vi "Read Task List.vi"(4 "Error In":errorcluster, 7 "Image Name":string) -> (0 "Error Out":errorcluster, 2 "Processes Found":i32, 3 "Processes":T1(array[cluster]))   [LabVIEW 2014, in "Managing Executables.lvlib"]
uses:
  Managing Executables.lvlib
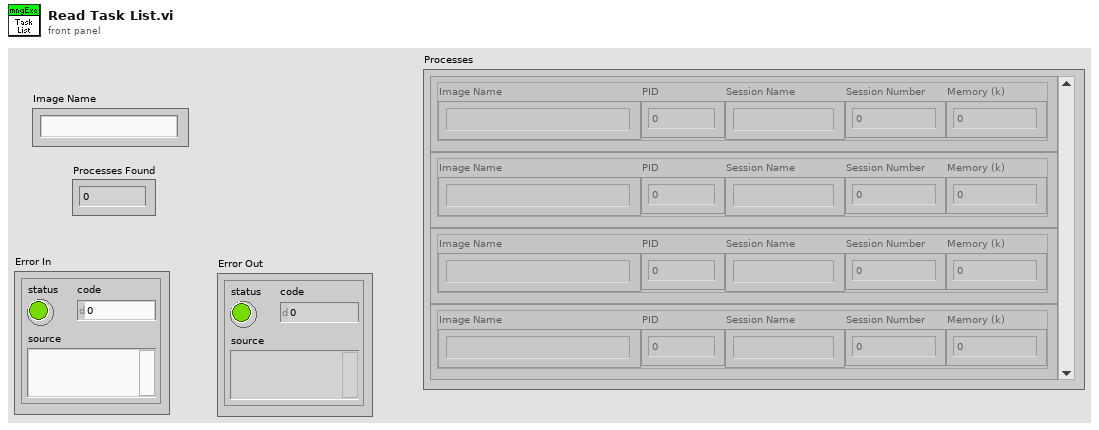
[diagram p1: front panel]
types:
  T1 = cluster{"Image Name":string, "PID":i32, "Session Name":string, "Session Number":i32, "Memory (k)":i32}[]
  T2 = cluster{"Image Name":string, "PID":i32, "Session Name":string, "Session Number":i32, "Memory (k)":i32}
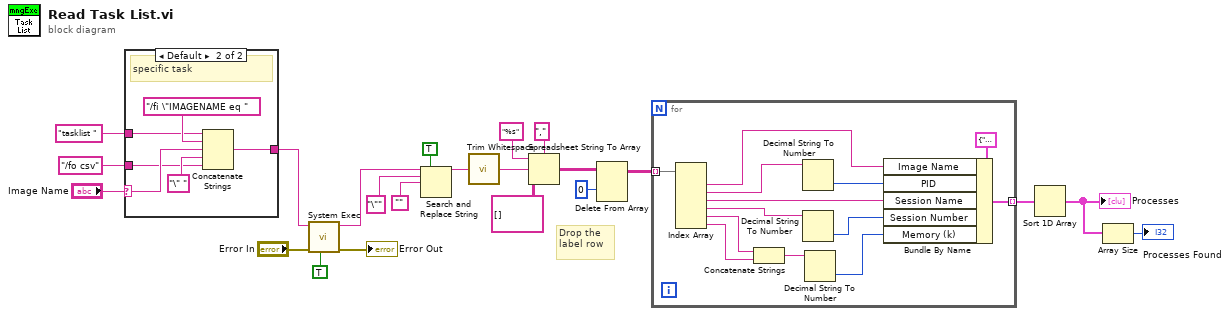
[diagram p0: block diagram]
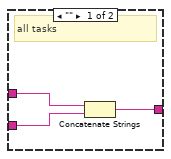
[diagram p2: hidden frame]
diagram:
  # "Drop the label row"
  n1 = case shown="Default" "Image Name" {
    selector: "Image Name" -> [_ w28]
    tunnel: [w23 w29] -> w7
    tunnel: "tasklist " -> [w25 w27]
    tunnel: "/fo csv" ("command line") -> [w24 w26]
    frame "" {
      # "all tasks"
      n2 = Concatenate Strings(w25, w24) -> (w23:string)
    }
    frame Default {
      # "specific task"
      n3 = Concatenate Strings(w27, "/fi \"IMAGENAME eq " ("command line"), w28, "\" " ("command line"), w26) -> (w29:string)
    }
  }
  n4 = call <vilib>:"System Exec.vi"("run minimized? (F)"=TRUE, "error in (no error)"="Error In", "command line"=w7) -> ("error out"=→"Error Out":errorcluster, "standard output"=w18:string)  [unwired: 5 in, 2 out]
  n5 = Search and Replace String(replace all?=TRUE ("replace all? (F)"), input string=w18, search string="\"", replace string="" ("search string")) -> (result string=w2:string)  [unwired: 4 in, 3 out]
  n6 = call <vilib>:"Trim Whitespace.vi"("string"=w2) -> ("trimmed string"=w3:string)  [unwired: 1 in]
  n7 = Spreadsheet String To Array(delimiter (Tab)=",", format string="%s", spreadsheet string=w3, array type (2D Dbl)=string[][] []) -> (array=w14:string[][])
  n8 = Delete From Array(array=w14, index (row)=0) -> (array with subset deleted=w12:string[][])  [unwired: 2 in, 1 out]
  n9 = for {
    tunnel: w12 -> [w42] mode=indexing
    tunnel: [w43] -> w9 mode=indexing
    n10 = Index Array(array=w42) -> (element #1=w34:string, element #2=w41:string, element #3=w39:string, element #4=w38:string, element #5=w35:string, element #6=w33:string)  [unwired: 6 in]
    n11 = Concatenate Strings(w35, w33) -> (w32:string)
    n12 = Decimal String To Number(string=w41) -> (number=w40:i32)  [unwired: 2 in, 1 out]
    n13 = Decimal String To Number(string=w38) -> (number=w37:i32)  [unwired: 2 in, 1 out]
    n14 = Decimal String To Number(string=w32) -> (number=w36:i32)  [unwired: 2 in, 1 out]
    n15 = Bundle By Name(cluster=T2 {"Image Name"="", "PID"=0, "Session Name"="", "Session Number"=0, "Memory (k)"=0}, "Image Name"=w34, "PID"=w40, "Session Name"=w39, "Session Number"=w37, "Memory (k)"=w36) -> (w43:T2)
  }
  n16 = Sort 1D Array(array=w9) -> (sorted array=w1:T1)
  "Processes" <- w1
  n17 = Array Size(array=w1) -> (size(s)=→"Processes Found":i32)
